vi "Create-log.vi"(8 "error in (no error)":errorcluster, 11 "Errors in":T1) -> (0 "error out":errorcluster, 3 "Errors out":T1)   [LabVIEW 2013, in "Error-handling.lvlib" / "Errors.lvclass"]
uses:
  Errors.lvclass
  Object-reference.ctl
  Errors.lvclass/Errors.ctl
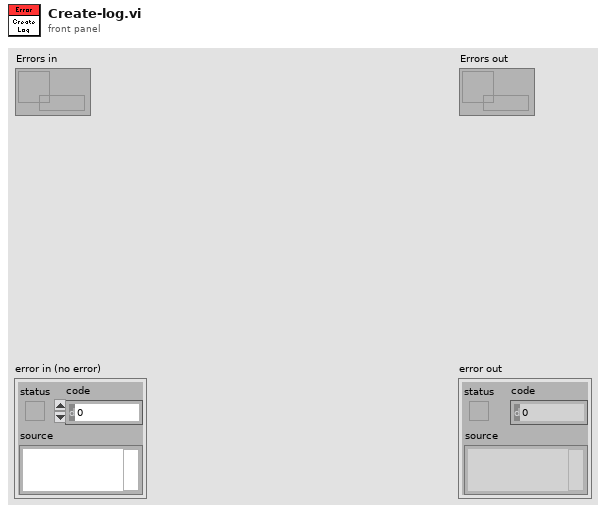
[diagram p1: front panel]
types:
  T1 = typedef "Error-handling.lvlib/Errors.lvclass/Object-reference.ctl" = refnum<data-value>
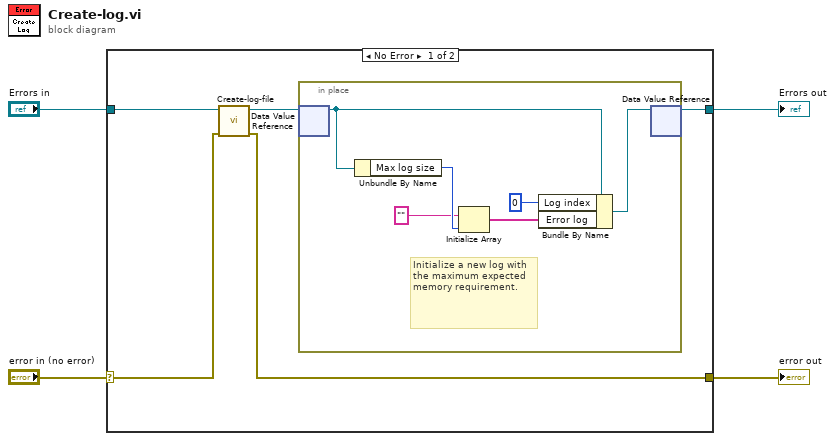
[diagram p0: block diagram]
diagram:
  n1 = case shown="No Error" "error in (no error)" {
    selector: "error in (no error)" -> [w8 w17]
    tunnel: [w7 w17] -> w3
    tunnel: [w5 w16] -> w1
    tunnel: "Errors in" -> [w9 w16]
    frame No Error {
      n2 = call "Create-log-file.vi"("error in (no error)"=w8, "Errors in"=w9) -> ("error out"=w7:errorcluster, "Errors out"=w6:T1)  [unwired: 8 in]
      n3 = in-place {
        # "Initialize a new log with the maximum expected memory requirement."
        n4 = in-place-dvr #1(w6) -> (w10:refnum<class "Errors.lvclass">)  [unwired: 1 out]
        n5 = Unbundle By Name(w10) -> ("Max log size"=w14:i32)
        n6 = Initialize Array("", w14) -> (w12:string[])
        n7 = Bundle By Name(cluster=w10, "Log index"=0, "Error log"=w12) -> (w11:refnum<class "Errors.lvclass">)
        n8 = in-place-dvr #1(w11) -> (w5:T1)  [unwired: 1 out]
      }
    }
    frame Error {
    }
  }
  "error out" <- w3
  "Errors out" <- w1
